vi "Programa_1.vi"() -> ()   [LabVIEW 2016]
panel:
  in  "file path (use dialog)":path
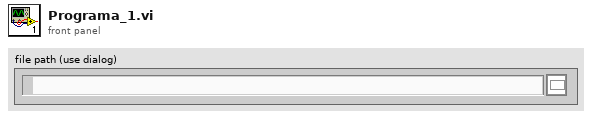
[diagram p1: front panel]
types:
  T1 = enum16{"open", "replace", "create", "open or create", "replace or create", "replace or create with confirmation"}
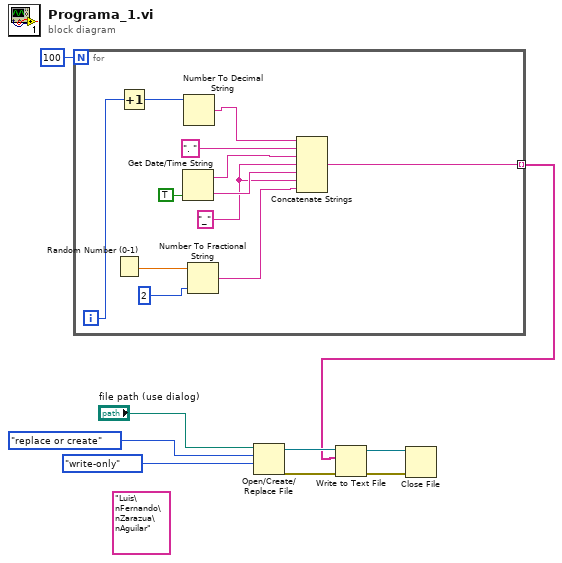
[diagram p0: block diagram]
diagram:
  (unwired) "Luis\nFernando\nZarazua\nAguilar" ("text")
  n1 = for {
    N: 100 -> [_]
    tunnel: [w15] -> w2 mode=indexing
    i -> [w13]
    w16 = "_" ("string")
    n2 = Random Number (0-1)() -> (number: 0 to 1=w12:dbl)
    n3 = Increment(x=w13) -> (x+1=w14:i32)
    n4 = Get Date/Time String(want seconds? (F)=TRUE) -> (date string=w19:string, time string=w17:string)  [unwired: 2 in]
    n5 = Number To Decimal String(number=w14) -> (decimal integer string=w21:string)  [unwired: 1 in]
    n6 = Number To Fractional String(number=w12, precision (6)=i16 2 ("width (-)")) -> (F-format string=w11:string)  [unwired: 2 in]
    n7 = Concatenate Strings(w21, ". " ("string"), w19, w16, w17, w16, w11) -> (w15:string)
  }
  n8 = Open/Create/Replace File(file path (use dialog)="file path (use dialog)", operation (0:open)=T1."replace or create", access (0:read/write)=enum16{"read/write", "read-only", "write-only"}."write-only") -> (refnum out=w8:refnum<file>, error out=w9:errorcluster)  [unwired: 3 in, 1 out]
  n9 = Write to Text File(file (use dialog)=w8, text=w2, error in=w9) -> (refnum out=w6:refnum<file>, error out=w7:errorcluster)  [unwired: 1 in, 1 out]
  n10 = Close File(refnum=w6, error in=w7) -> ()  [unwired: 2 out]
